vi "Write Event.vi"(8 "error in (no error)":errorcluster, 10 "Event":refnum<class "Event.lvclass">, 11 "EventMgr in":refnum<class "EventMgr.lvclass">) -> (0 "error out":errorcluster, 3 "EventMgr out":refnum<class "EventMgr.lvclass">)   [LabVIEW 2013, in "EventMgr.lvclass"]
uses:
  EventMgr.lvclass
  Utilities/Event/Event.lvclass
  EventMgr.lvclass/EventMgr.ctl
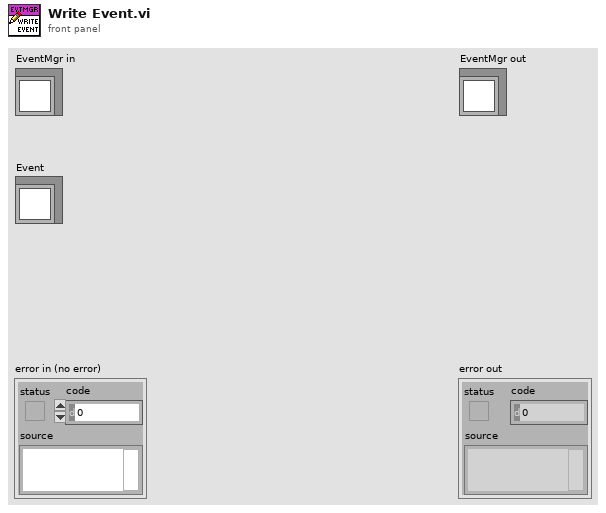
[diagram p1: front panel]
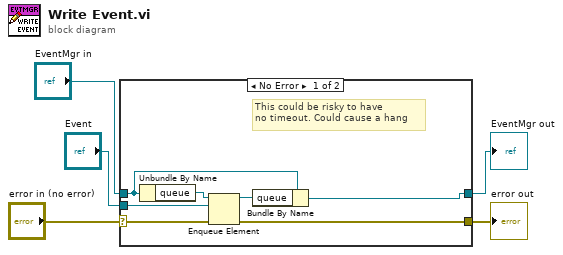
[diagram p0: block diagram]
diagram:
  n1 = case shown="No Error" "error in (no error)" {
    selector: "error in (no error)" -> [w7 w14]
    tunnel: [w6 w14] -> w4
    tunnel: [w9 w13] -> w2
    tunnel: "EventMgr in" -> [w12 w13]
    tunnel: "Event" -> [w10 _]
    frame No Error {
      # "This could be risky to have \nno timeout. Could cause a hang"
      n2 = Unbundle By Name(w12) -> ("queue"=w11:refnum<queue>)
      n3 = Enqueue Element(queue=w11, element=w10, error in (no error)=w7) -> (queue out=w8:refnum<queue>, error out=w6:errorcluster)  [unwired: 1 in, 1 out]
      n4 = Bundle By Name(cluster=w12, "queue"=w8) -> (w9:refnum<class "EventMgr.lvclass">)
    }
    frame Error {
    }
  }
  "error out" <- w4
  "EventMgr out" <- w2
